vi "Constructor.vi"(8 "error in (no error)":errorcluster, 11 "SerDes in":refnum<class "OOPbyRef.lvclass">) -> (0 "error out":errorcluster, 3 "SerDes out":refnum<class "OOPbyRef.lvclass">)   [LabVIEW 2021, in "DQMH_byOOPRef.lvlib" / "OOPbyRef.lvclass"]
uses:
  OOPbyRef.lvclass
  OOPbyRef.lvclass/OOPbyRef.ctl
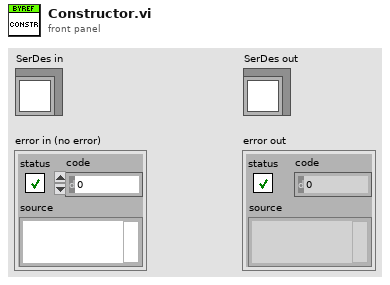
[diagram p1: front panel]
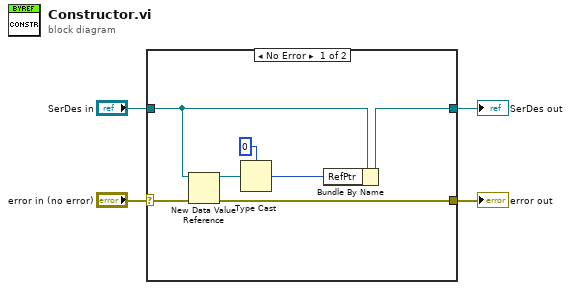
[diagram p0: block diagram]
diagram:
  n1 = case shown="No Error" "error in (no error)" {
    selector: "error in (no error)" -> [w6 w13]
    tunnel: [w5 w13] -> w3
    tunnel: [w8 w12] -> w1
    tunnel: "SerDes in" -> [w11 w12]
    frame No Error {
      n2 = New Data Value Reference(data value=w11, error in=w6) -> (data value reference=w9:refnum<data-value>, error out=w5:errorcluster)
      n3 = Type Cast(type=0, x=w9) -> (*(type *) &x=w7:i32)
      n4 = Bundle By Name(cluster=w11, "RefPtr"=w7) -> (w8:refnum<class "OOPbyRef.lvclass">)
    }
    frame Error {
    }
  }
  "error out" <- w3
  "SerDes out" <- w1
